vi "Login Success.vi"(8 "error in (no error)":errorcluster, 10 "username":string, 11 "[User] Userinfo Binary in":refnum<class "[User] Userinfo Binary.lvclass">) -> (0 "error out":errorcluster, 3 "[User] Userinfo Binary out":refnum<class "[User] Userinfo Binary.lvclass">)   [LabVIEW 2020, in "[User] Userinfo Binary.lvclass"]
uses:
  [User] Userinfo Binary.lvclass
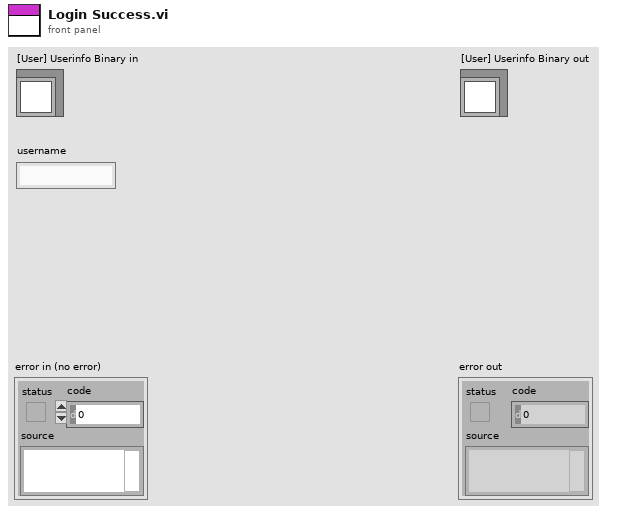
[diagram p1: front panel]
types:
  T1 = typedef "[User] Userinfo Binary.lvclass/userinfo.ctl" = cluster{"password":string, "authority":i8, "department":string, "post":string, "remark":string, "create time":timestamp, "last login time":timestamp}
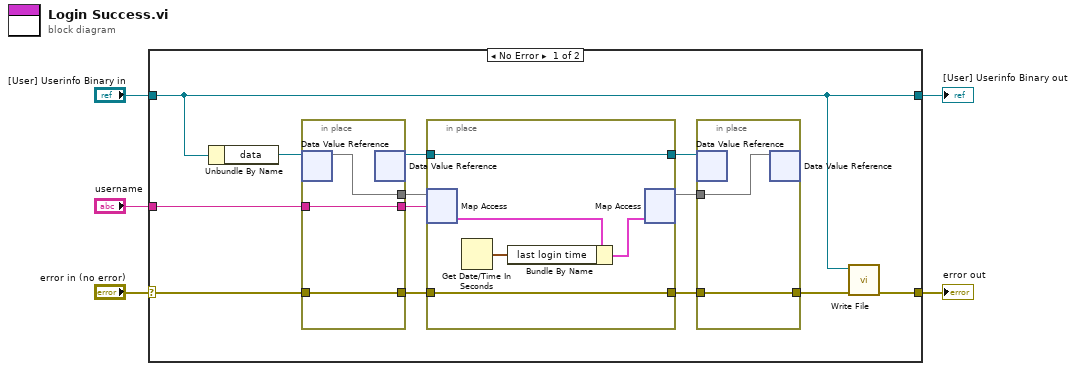
[diagram p0: block diagram]
diagram:
  n1 = case shown="No Error" "error in (no error)" {
    selector: "error in (no error)" -> [w18 w30]
    tunnel: [w6 w30] -> w4
    tunnel: "[User] Userinfo Binary in" -> [w7 w29]
    tunnel: [w7 w29] -> w2
    tunnel: "username" -> [w16 _]
    frame No Error {
      n2 = Unbundle By Name(w7) -> ("data"=w17:refnum<data-value>)
      n3 = in-place {
        in-place-border: w18 -> [w28]
        in-place-border: [w28] -> w13
        in-place-border: [w27] -> w15
        in-place-border: w16 -> [w26]
        in-place-border: [w26] -> w14
        n4 = in-place-dvr #1(w17) -> (w27:map{string, T1})  [unwired: 1 out]
        n5 = in-place-dvr #1() -> (w11:refnum<data-value>)  [unwired: 1 in, 1 out]
      }
      n6 = in-place {
        in-place-border: w13 -> [w22]
        in-place-border: [w22] -> w12
        in-place-border: w11 -> [w21]
        in-place-border: [w21] -> w10
        n7 = in-place-map #2(w15, w14) -> (w25:T1)  [unwired: 1 in, 1 out]
        n8 = Get Date/Time In Seconds() -> (seconds since 1Jan1904=w24:timestamp)
        n9 = Bundle By Name(cluster=w25, "last login time"=w24) -> (w23:T1)
        n10 = in-place-map #2(w23) -> (w9:map{string, T1})  [unwired: 1 in, 2 out]
      }
      n11 = in-place {
        in-place-border: w12 -> [w20]
        in-place-border: [w20] -> w8
        in-place-border: w9 -> [w19]
        n12 = in-place-dvr #3(w10) -> ()  [unwired: 2 out]
        n13 = in-place-dvr #3(w19) -> ()  [unwired: 2 out]
      }
      n14 = call "Write File.vi"("error in (no error)"=w8, "[User] Userinfo Binary in"=w7) -> ("error out"=w6:errorcluster)  [unwired: 8 in, 1 out]
    }
    frame Error {
    }
  }
  "error out" <- w4
  "[User] Userinfo Binary out" <- w2
